vi "UpdateSpotMap.vi"(0 "Rawdata":T1, 1 "Coefficients":dbl[][](array[numeric]) format="%.2f", 2 "Mask (input)":T1, 3 "Display Input":T1, 4 "radius":i32, 5 "error in (no error)":errorcluster) -> (6 "Mask (output)":T1, 7 "Display (output":T1, 8 "error out":errorcluster)   [LabVIEW 2009]
uses:
  <vilib>/vision/Image Controls.llb/IMAQ Image.ctl
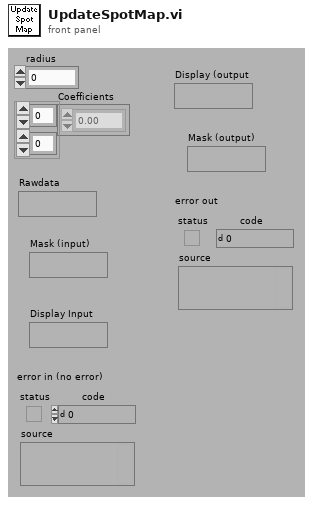
[diagram p1: front panel]
types:
  T1 = typedef "IMAQ Image.ctl" = refnum<image>
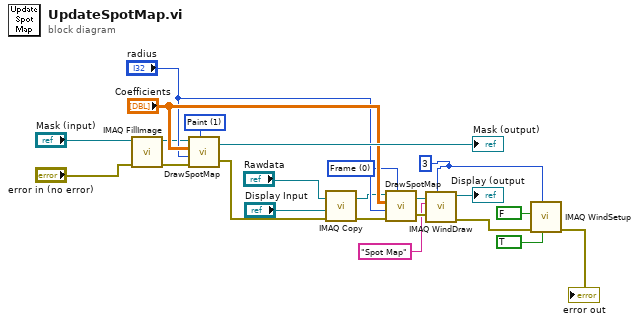
[diagram p0: block diagram]
diagram:
  w2 = 3 ("Window Number (0...15)")
  w11 = u16 1 items=["Frame", "Paint", "Invert Frame", "Invert Paint"] ("Draw Mode")
  w12 = u16 0 items=["Frame", "Paint", "Invert Frame", "Invert Paint"] ("Draw Mode")
  n1 = call "IMAQ FillImage"("error in (no error)"="error in (no error)", "Image"="Mask (input)") -> ("error out"=w18:errorcluster, "Image Out"=w19:T1)  [unwired: 8 in]
  n2 = call "DrawSpotMap.vi"("Draw Mode"=w11, "error in (no error)"=w18, "radius"="radius", "Coefficients (2D)"="Coefficients", "Image Dst"=w19) -> ("error out"=w9:errorcluster, "Spot Map"=→"Mask (output)":T1)  [unwired: 1 in]
  n3 = call "IMAQ Copy"("error in (no error)"=w9, "Image Dst"="Display Input", "Image Src"="Rawdata") -> ("error out"=w13:errorcluster, "Image Dst Out"=w1:T1)  [unwired: 3 in]
  n4 = call "DrawSpotMap.vi"("Draw Mode"=w12, "error in (no error)"=w13, "radius"="radius", "Coefficients (2D)"="Coefficients", "Image Dst"=w1) -> ("error out"=w15:errorcluster, "Spot Map"=w3:T1)  [unwired: 1 in]
  n5 = call "IMAQ WindDraw"("Window Number (0...15)"=w2, "error in (no error)"=w15, "Title"="Spot Map", "Image"=w3) -> ("error out"=w8:errorcluster, "Image Out (duplicate)"=→"Display (output":T1)  [unwired: 6 in]
  n6 = call "IMAQ WindSetup"("Window is floating? (No)"=TRUE, "Window Number (0...15)"=w2, "error in (no error)"=w8, "Window can close? (Yes)"=FALSE) -> ("error out"=→"error out":errorcluster)  [unwired: 7 in]
